vi "Build Read Parameters.vi"(4 "TypeMap in":refnum<class "TypeMap.lvclass">, 8 "error in (no error)":errorcluster, 10 "object":variant, 11 "SqlMapper in":refnum<class "SqlMapper.lvclass">) -> (0 "error out":errorcluster, 1 "DynamicParameters out":refnum<class "DynamicParameters.lvclass">, 3 "SqlMapper out":refnum<class "SqlMapper.lvclass">)   [LabVIEW 2020, in "ORM.lvlib" / "TypeMap.lvclass"]
uses:
  TypeMap.lvclass
  DynamicParameters/DynamicParameters.lvclass
  SqlMapper/SqlMapper.lvclass
  TypeMap.lvclass/TypeMap.ctl
  DynamicParameters/DynamicParameters.lvclass/DynamicParameters.ctl
  DynamicParameters/Write KeyProperties.vi
  Read Autokey.vi
  Read KeyProperties.vi
  <vilib>/Utility/error.llb/Error Cluster From Error Code.vi
  <vilib>/ErrorRing/Error Ring.xnode
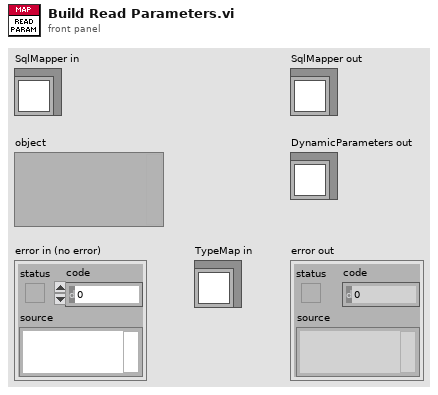
[diagram p1: front panel]
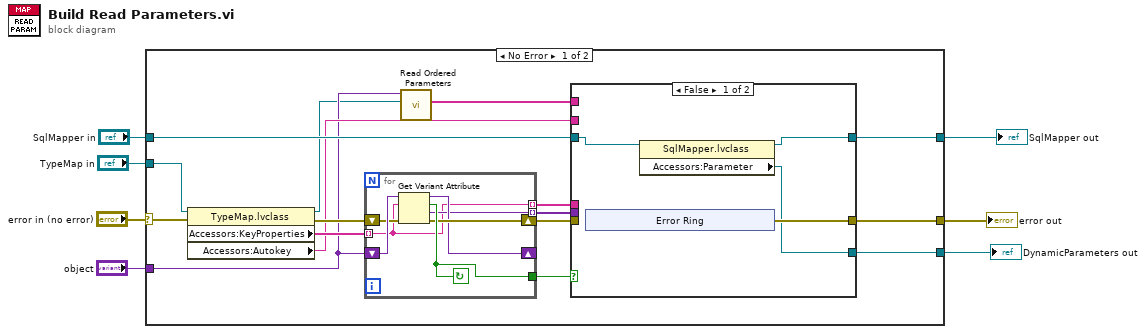
[diagram p0: block diagram]
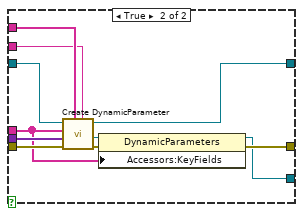
[diagram p2: hidden frame]
diagram:
  n1 = case shown="No Error" "error in (no error)" {
    selector: "error in (no error)" -> [w21 w51]
    tunnel: "TypeMap in" -> [w20 _]
    tunnel: "object" -> [w10 _]
    tunnel: "SqlMapper in" -> [w16 w52]
    tunnel: [w14 w52] -> w3
    tunnel: [w13 w51] -> w2
    tunnel: [w12 _] -> w1
    frame No Error {
      n2 = property class="TypeMap.lvclass"(reference=w20, error in=w21) -> (reference out=w8:refnum<class "TypeMap.lvclass">, error out=w22:errorcluster, "Accessors:KeyProperties"=w23:string[], "Accessors:Autokey"=w11:string)
      n3 = for {
        tunnel: w23 -> [w44] mode=indexing
        tunnel: [w49] -> w15
        shift-right: [w48] -> w19
        shift-left: w22 -> [w47]
        shift-right: [w46] -> _
        shift-left: w10 -> [w50]
        tunnel: [w45] -> w18 mode=indexing
        tunnel: [w44] -> w17 mode=indexing
        stop <- w49 continue-if-true
        n4 = Get Variant Attribute(Variant=w50, name=w44, error in=w47) -> (duplicate Variant=w46:variant, found=w49:bool, value=w45:variant, error out=w48:errorcluster)  [unwired: 1 in]
      }
      n5 = call "Read Ordered Parameters.vi"("TypeMap in"=w8, "Object In"=w10) -> ("Fields"=w9:string[])  [unwired: 6 in, 3 out]
      n6 = case shown="False" w15 {
        tunnel: w19 -> [_ w43]
        tunnel: w18 -> [_ w42]
        tunnel: w17 -> [_ w33]
        tunnel: w16 -> [w26 w41]
        tunnel: [w24 w40] -> w14
        tunnel: [w27 w36] -> w13
        tunnel: [w25 w34] -> w12
        tunnel: w9 -> [_ w38]
        tunnel: w11 -> [_ w37]
        frame False {
          n7 = xnode "Error Ring"() -> ("error out"=w27:errorcluster)
          n8 = property class="SqlMapper.lvclass"(reference=w26) -> (reference out=w24:refnum<class "SqlMapper.lvclass">, "Accessors:Parameter"=w25:refnum<class "DynamicParameters.lvclass">)  [unwired: 1 in, 1 out]
        }
        frame True {
          n9 = call "Create DynamicParameter.vi"("AutoKey"=w37, "RequestedFields"=w38, "error in (no error)"=w43, "ParameterValues"=w42, "ParameterNames"=w33, "SqlMapper in"=w41) -> ("error out"=w39:errorcluster, "Parameters"=w35:refnum<class "DynamicParameters.lvclass">, "SqlMapper out"=w40:refnum<class "SqlMapper.lvclass">)  [unwired: 1 in, 2 out]
          n10 = property class="DynamicParameters"(reference=w35, error in=w39, "Accessors:KeyFields"=w33) -> (reference out=w34:refnum<class "DynamicParameters.lvclass">, error out=w36:errorcluster)
        }
      }
    }
    frame Error {
    }
  }
  "error out" <- w2
  "SqlMapper out" <- w3
  "DynamicParameters out" <- w1
